vi "CRON.CreateRequests.vi"(8 "error in (no error)":errorcluster) -> (0 "error out":errorcluster, 3 "Requests":T1)   [LabVIEW 2024, in "CRON.lvclass"]
uses:
  CRON.lvclass
  CRON.lvclass/CRON.ctl
  Request Events--cluster.ctl
  Do Something Args.ctl
  RQMHCore/ModuleCore/Reply.ctl
  RQMHCore/ModuleCore/Module.lvclass
  <vilib>/LabVIEW Open Source Project/Cron Scheduler/Cron/Cron.lvclass
  Set Schedule Args.ctl
  Arm Args.ctl
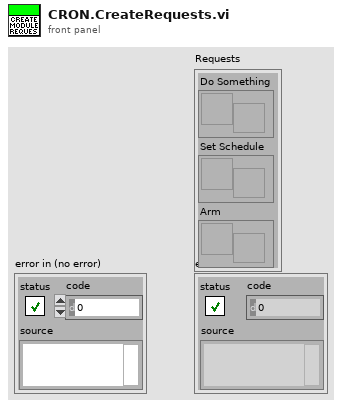
[diagram p1: front panel]
types:
  T1 = typedef "CRON.lvclass/Request Events--cluster.ctl" = cluster{"Do Something":refnum<user-event>, "Set Schedule":refnum<user-event>, "Arm":refnum<user-event>}
  T2 = typedef "CRON.lvclass/Arm Args.ctl" = cluster{"null":bool}
  T3 = typedef "Module.lvclass/Reply.ctl" = cluster{"Expects Reply":bool, "Reply":refnum<notifier>}
  T4 = typedef "CRON.lvclass/Set Schedule Args.ctl" = cluster{"Cron":refnum<class "Cron.lvclass">}
  T5 = typedef "CRON.lvclass/Do Something Args.ctl" = cluster{"Msg":string}
  T6 = cluster{"Do Something Args":T5, "Reply Payload":T3}
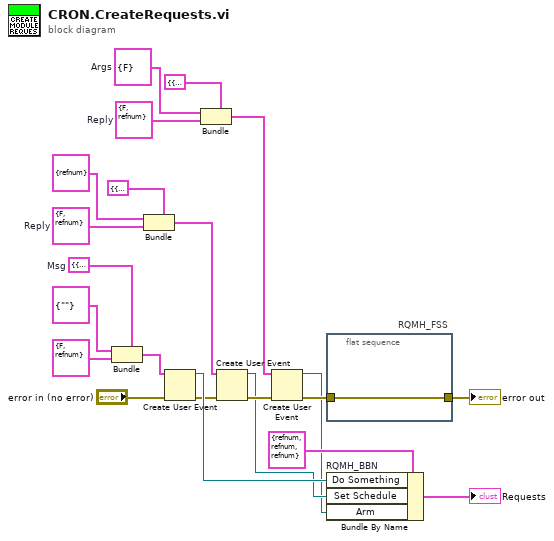
[diagram p0: block diagram]
diagram:
  w2 = T2 {"null"=FALSE}  # Args
  w3 = T3 {"Expects Reply"=FALSE, "Reply"=refnum}  # Reply
  w9 = T3 {"Expects Reply"=FALSE, "Reply"=refnum}  # Reply
  w16 = T6 {"Do Something Args"={"Msg"=""}, "Reply Payload"={"Expects Reply"=FALSE, "Reply"=refnum}}  # Msg
  n1 = Bundle(cluster=w16, "Do Something Args"=T5 {"Msg"=""}, "Reply Payload"=T3 {"Expects Reply"=FALSE, "Reply"=refnum}) -> (w19:T6)
  n2 = Bundle(cluster=cluster{"Args":T4, "Reply":T3} {"Args"={"Cron"=refnum}, "Reply"={"Expects Reply"=FALSE, "Reply"=refnum}} ("Msg"), "Args"=T4 {"Cron"=refnum} ("Set Schedule Args"), "Reply"=w9) -> (w10:cluster{"Args":T4, "Reply":T3})
  n3 = Create User Event(user event datatype=w19, error in="error in (no error)") -> (user event=w15:refnum<user-event>, error out=w13:errorcluster)
  n4 = Bundle(cluster=cluster{"Args":T2, "Reply":T3} {"Args"={"null"=FALSE}, "Reply"={"Expects Reply"=FALSE, "Reply"=refnum}} ("Msg"), "Args"=w2, "Reply"=w3) -> (w4:cluster{"Args":T2, "Reply":T3})
  n5 = Create User Event(user event datatype=w10, error in=w13) -> (user event=w11:refnum<user-event>, error out=w12:errorcluster)
  n6 = Create User Event(user event datatype=w4, error in=w12) -> (user event=w5:refnum<user-event>, error out=w6:errorcluster)
  n7 = flat-sequence "RQMH_FSS" {
    tunnel: [w23] -> w14
    tunnel: w6 -> [w23]
    frame #0 {
    }
  }
  n8 = Bundle By Name "RQMH_BBN"(cluster=T1 {"Do Something"=refnum, "Set Schedule"=refnum, "Arm"=refnum} ("Requests"), "Do Something"=w15, "Set Schedule"=w11, "Arm"=w5) -> (→"Requests":T1)
  "error out" <- w14
